vi "ReadObjectLayout.vi"(7 "properties to ignore":variant, 8 "error in (no error)":errorcluster, 10 "GObj Refnum":refnum<vi>, 11 "Splitter Layout in":refnum<class "Splitter Layout.lvclass">) -> (0 "error out":errorcluster, 3 "Splitter Layout out":refnum<class "Splitter Layout.lvclass">)   [LabVIEW 2010, in "NI_SE_Front Panel Layout.lvlib" / "Splitter Layout.lvclass"]
doc: "Read layout information from the GObj Refnum."
uses:
  Splitter Layout.lvclass
  Object Layout/Object Layout.lvclass
  Splitter Layout.lvclass/Splitter Layout.ctl
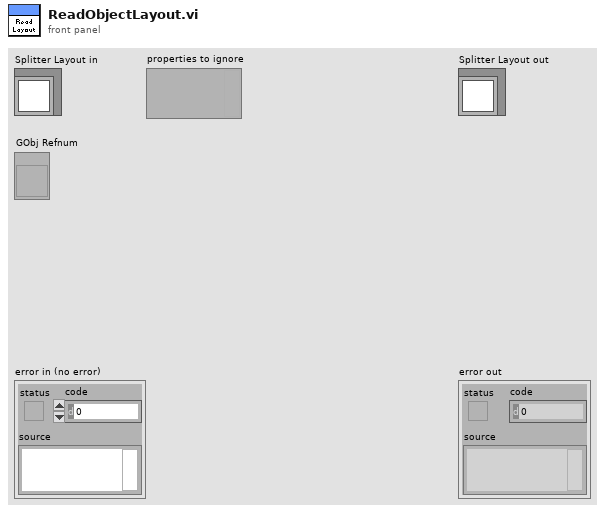
[diagram p1: front panel]
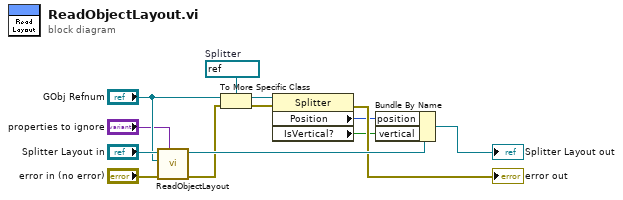
[diagram p0: block diagram]
diagram:
  w5 = refnum<vi> refnum  # Splitter
  n1 = call-parent "ReadObjectLayout.vi"("properties to ignore"="properties to ignore", "error in (no error)"="error in (no error)", "GObj Refnum"="GObj Refnum", "Object Layout in"="Splitter Layout in") -> ("error out"=w10:errorcluster, "Object Layout out"=w11:refnum<class "Splitter Layout.lvclass">)  [unwired: 6 in]
  n2 = To More Specific Class(target class=w5, reference="GObj Refnum", error in=w10) -> (specific class reference=w4:refnum<vi>, error out=w3:errorcluster)
  n3 = property class="Splitter"(reference=w4, error in=w3) -> (error out=→"error out":errorcluster, "Position"=w2:i32, "IsVertical?"=w1:bool)  [unwired: 1 out]
  n4 = Bundle By Name(cluster=w11, "position"=w2, "vertical"=w1) -> (→"Splitter Layout out":refnum<class "Splitter Layout.lvclass">)
